vi "Get System Environment Variable.vi"(3 "Environment Variable Name":string="COMPUTERNAME") -> (1 "Value":string)   [LabVIEW 2017]
uses:
  kernel32.dll
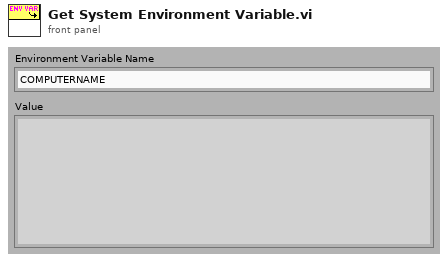
[diagram p1: front panel]
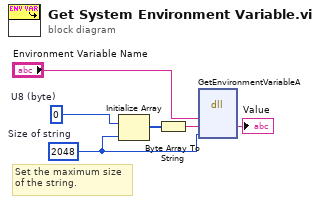
[diagram p0: block diagram]
diagram:
  w3 = u8 0  # U8 (byte)
  w4 = 2048  # Size of string
  # "Set the maximum size\nof the string."
  n1 = Initialize Array(w3, w4) -> (w2:u8[])
  n2 = Byte Array To String(unsigned byte array=w2) -> (string=w1:string)
  n3 = dll-call lib="kernel32.dll" fn="GetEnvironmentVariableA"("EnvVarName"="Environment Variable Name", "lpBuffer"=w1, "namelength"=w4) -> ("lpBuffer"=→"Value":string)  [unwired: 6 in, 2 out]
